vi "VisualizeCHROMADC.vi"() -> ()   [LabVIEW 2018, in "Visualization.lvlib" / "VisualizeAcPwr.lvclass"]
uses:
  VisualizeAcPwr.lvclass
  <vilib>/event_ctls.llb/usereventprio.ctl
  VisualizeBase/VisualizeBase_class/Requests/clUserEventType.ctl
  <vilib>/Utility/error.llb/Error Cluster From Error Code.vi
  <vilib>/ErrorRing/Error Ring.xnode
  VisualizeBase/VisualizeBase_class/VisualizeBase.lvclass
  <userlib>/NIST/NISTErrorLib/NISTErrorLib.lvlib
  AcPwr/AcPwrModule/AcPwrModule.lvlib
panel:
  in  "GraphAxis":u32[](array[numeric])=[0, 1, 1] max=1
  out "Chroma DC":waveform(dbl)[](graph)
  out "ErrorArray":errorcluster[](array[cluster])
  in  "QueuName":string="CHROMADCVQ"
  in  "btnStop":bool
  in  "btnReset":bool
  in  "btnClear":bool
  # "0=Left and 1=Right"
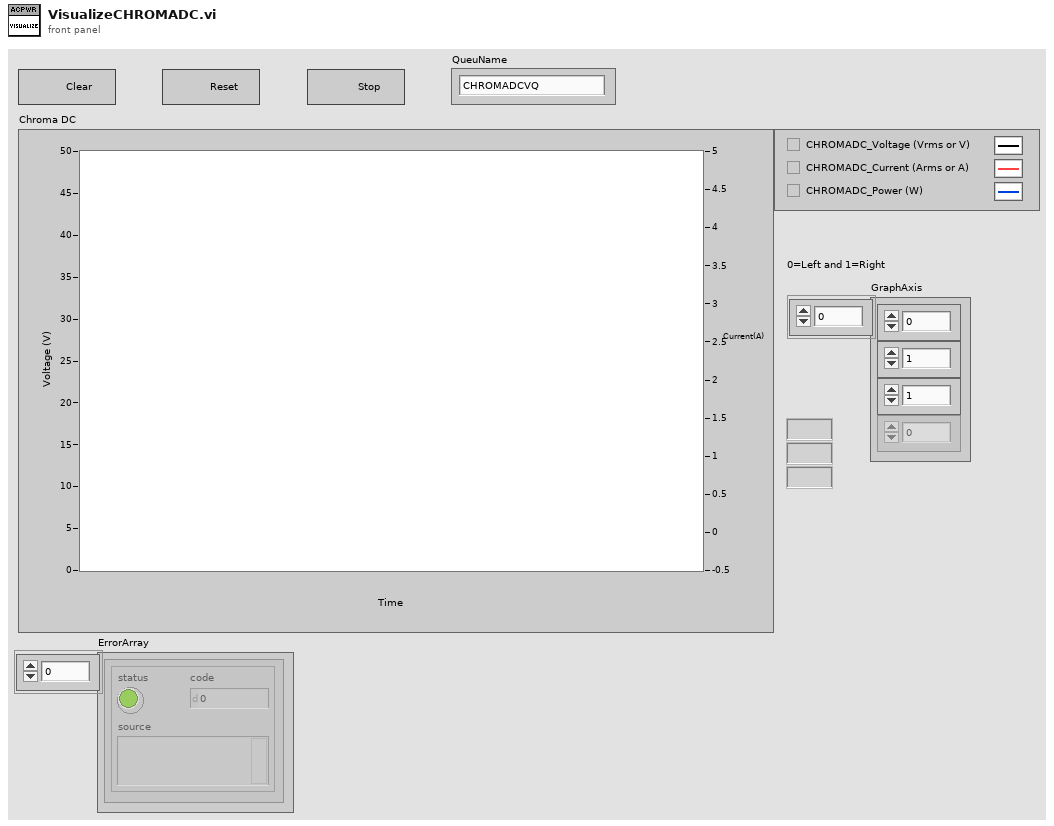
[diagram p1: front panel]
types:
  T1 = typedef "Visualization.lvlib/VisualizeBase.lvclass/clRequestEvents.ctl" = cluster{"StopRequest":refnum<user-event>, "ResetRequest":refnum<user-event>}
  T2 = typedef "AcPwrModule.lvlib/clBroadcastEvents.ctl" = cluster{"DidInit":refnum<user-event>, "StatusUpdate":refnum<user-event>, "ErrorReport":refnum<user-event>, "DidStop":refnum<user-event>, "PathToINI":refnum<user-event>, "Measurements":refnum<user-event>, "LoadConfigFile":refnum<user-event>}
  T3 = typedef "Visualization.lvlib/VisualizeBase.lvclass/clUserEventType.ctl" = cluster{"BusIndex":i8, "Data":variant}
  T4 = typedef "usereventprio.ctl" = enum32{"high priority", "normal priority"}
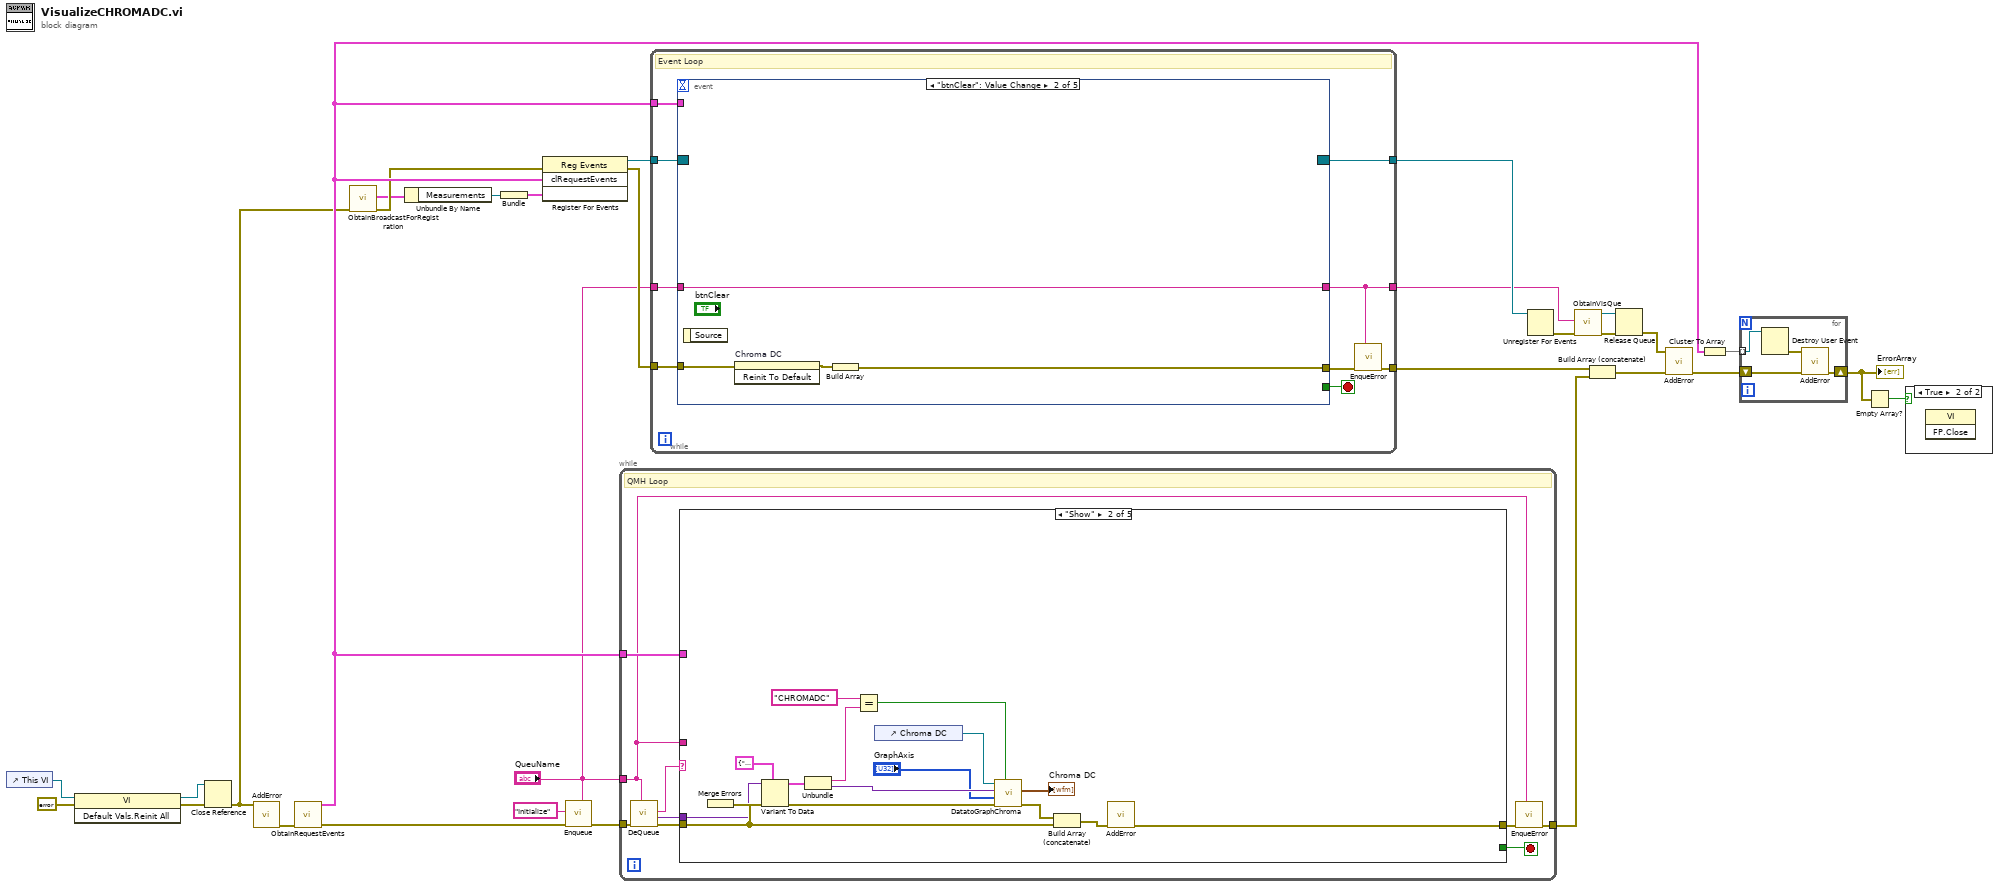
[diagram p0: block diagram]
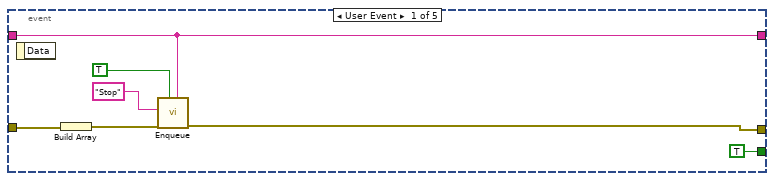
[diagram p3: hidden frame]
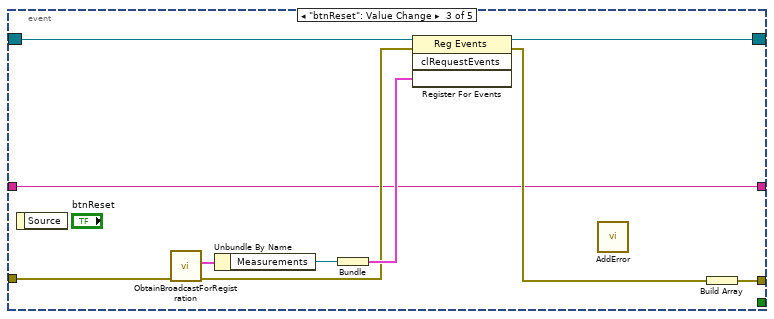
[diagram p4: hidden frame]
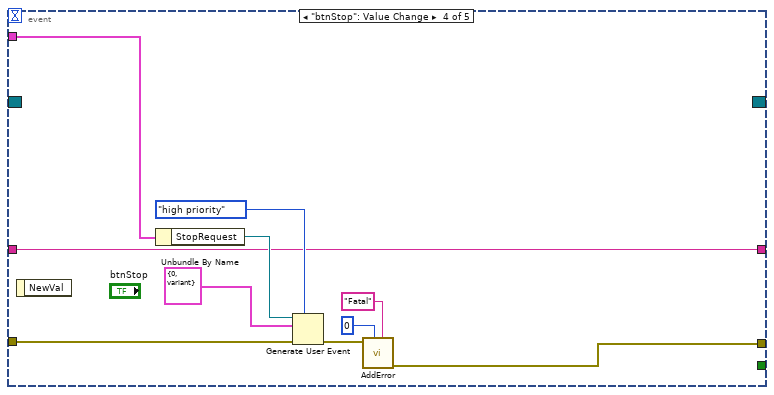
[diagram p5: hidden frame]
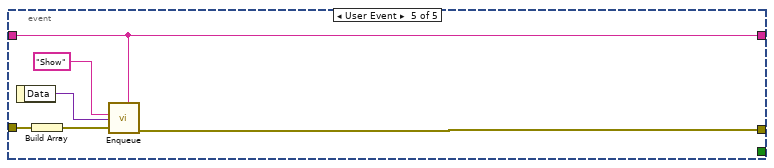
[diagram p6: hidden frame]
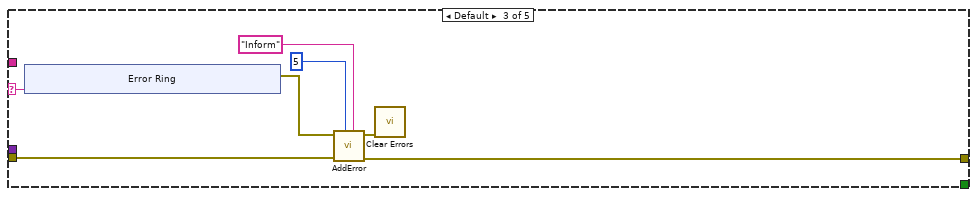
[diagram p8: hidden frame]
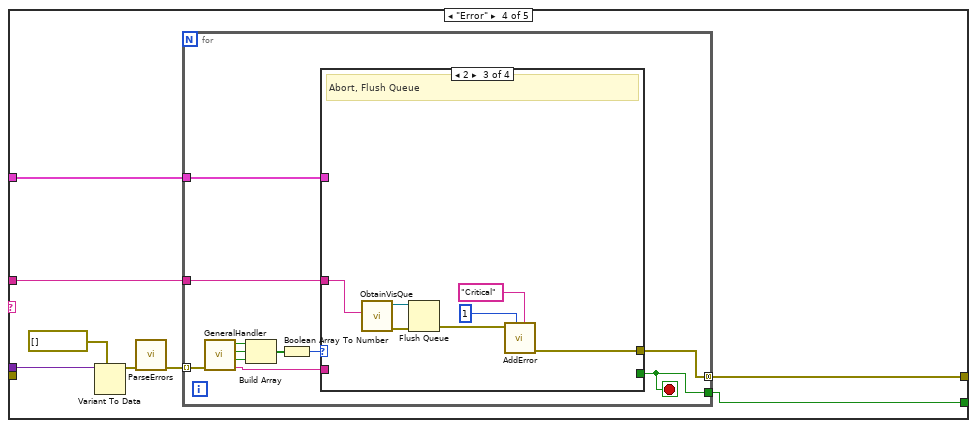
[diagram p9: hidden frame]
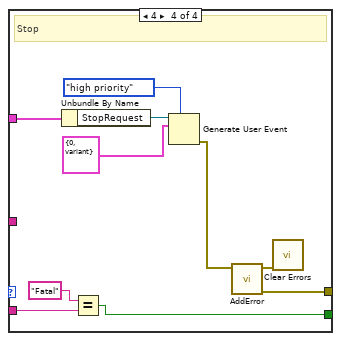
[diagram p12: hidden frame]
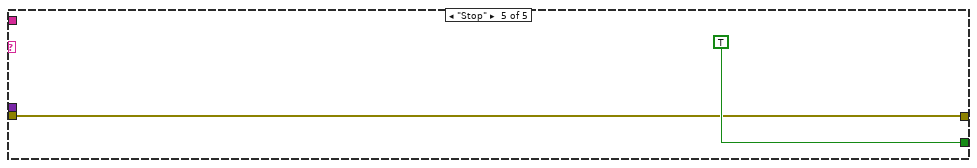
[diagram p13: hidden frame]
diagram:
  n1 = control-ref of="This VI"() -> (w10:refnum<vi>)
  n2 = invoke class="VI" method="Default Vals.Reinit All"(reference=w10, error in=errorcluster {"status"=FALSE, "code"=0, "source"=""} ("error in (no error)")) -> (reference out=w7:refnum<vi>, error out=w8:errorcluster)  [unwired: 1 in, 1 out]
  n3 = Close Reference(reference=w7, error in (no error)=w8) -> (error out=w5:errorcluster)
  n4 = call <userlib>:"AddError.vi"("error in (no error)"=w5) -> ("ErrorArray"=w27:errorcluster[])  [unwired: 9 in, 1 out]
  n5 = call "ObtainRequestEvents.vi"("Error"=w27) -> ("Error"=w12:errorcluster[], "clRequestEvents"=w16:T1)  [unwired: 9 in]
  n6 = call "ObtainBroadcastForRegistration.vi"("error in (no error)"=w5) -> ("error out"=w4:errorcluster, "clBroadcastEvents"=w3:T2)  [unwired: 9 in]
  n7 = Unbundle By Name(w3) -> ("Measurements"=w14:refnum<user-event>)
  n8 = Bundle("Measurements"=w14) -> (w13:cluster{"Measurements":refnum<user-event>})  [unwired: 1 in]
  n9 = register-events(error in=w4, w16, w13) -> (reference out=w28:refnum<event-registration>, error out=w11:errorcluster)  [unwired: 1 in]
  n10 = call "Enqueue.vi"("QueName"="QueuName", "Error"=w12, "Message"="Initialize") -> ("Error"=w29:errorcluster[])  [unwired: 8 in]
  n11 = while {
    tunnel: w29 -> [w39]
    tunnel: [w33] -> w23
    tunnel: "QueuName" -> [w31]
    tunnel: w16 -> [w32]
    stop <- w34 stop-if-true
    # "QMH Loop"
    n12 = call "DeQueue.vi"("QueName"=w31, "Error"=w39) -> ("Error"=w36:errorcluster[], "Data"=w37:variant, "Message"=w38:string)  [unwired: 7 in]
    n13 = case shown="\"Show\"" w38 {
      selector: w38 -> [_ _ w63 _ _]
      tunnel: w37 -> [_ w49 _ w78 _]
      tunnel: w36 -> [w40 w55 w61 _ w107]
      tunnel: [w40 w56 w60 w74 w107] -> w35
      tunnel: [_ _ _ w73 TRUE] -> w34
      tunnel: w32 -> [_ _ _ w72 _]
      tunnel: w31 -> [_ _ _ w71 _]
      frame "Initialize" {
      }
      frame "Show" {
        n14 = Merge Errors(w55) -> (w48:errorcluster)
        n15 = Variant To Data(error in=w48, type=cluster{string, "Data":variant} {"", "Data"=variant}, Variant=w49) -> (data=w50:cluster{string, "Data":variant}, error out=w45:errorcluster)
        n16 = Unbundle(w50) -> (w47:string, "Data"=w46:variant)
        n17 = Equal?(x="CHROMADC", y=w47) -> (x = y?=w43:bool)
        n18 = control-ref of="Chroma DC"() -> (w52:refnum<vi>)
        n19 = call "DatatoGraphChroma.vi"("Boolean"=w43, "error in (no error)"=w45, "Array 2"="GraphAxis", "Data"=w46, "WaveformChart in"=w52) -> ("error out"=w42:errorcluster, "Array"=→"Chroma DC":waveform(dbl)[])  [unwired: 3 in, 2 out]
        n20 = Build Array (concatenate)(w42, w55) -> (w54:errorcluster[])
        n21 = call <userlib>:"AddError.vi"("ErrorArray"=w54) -> ("ErrorArray"=w56:errorcluster[])  [unwired: 9 in, 1 out]
      }
      frame Default {
        n22 = xnode "Error Ring"("parameter 0"=w63) -> ("error out"=w62:errorcluster)
        n23 = call <userlib>:"AddError.vi"("Severity"="Inform" ("String"), "Priority"=u8 5, "ErrorArray"=w61, "error in (no error)"=w62) -> ("ErrorArray"=w60:errorcluster[], "error out"=w59:errorcluster)  [unwired: 6 in]
        n24 = call <vilib>:"Clear Errors.vi"("error in (no error)"=w59) -> ()  [unwired: 5 in, 2 out]
      }
      frame "Error" {
        n25 = Variant To Data(type=errorcluster[] [], Variant=w78) -> (data=w76:errorcluster[])  [unwired: 1 in, 1 out]
        n26 = call <userlib>:"ParseErrors.vi"("ErrorArray"=w76) -> ("ErrorArray"=w75:errorcluster[])  [unwired: 8 in, 2 out]
        n27 = for {
          tunnel: w75 -> [w89] mode=indexing
          tunnel: [w83] -> w74 mode=concatenating
          tunnel: [w81] -> w73
          tunnel: w72 -> [w80]
          tunnel: w71 -> [w79]
          stop <- w81 stop-if-true
          n28 = call <userlib>:"GeneralHandler.vi"("error in (no error)"=w89) -> ("Severity"=w82:string, "Stop"=w86:bool, "Abort"=w87:bool, "Continue"=w88:bool)  [unwired: 7 in]
          n29 = Build Array(w88, w87, w86) -> (w85:bool[])
          n30 = Boolean Array To Number(Boolean array=w85) -> (number=w84:u32)
          n31 = case shown="2" w84 {
            tunnel: [_ _ w94 w105] -> w83
            tunnel: w82 -> [_ _ _ w100]
            tunnel: [_ _ _ w98] -> w81
            tunnel: w80 -> [_ _ _ w97]
            tunnel: w79 -> [_ _ w90 _]
            frame 0, Default {
              # "No Dialog"
            }
            frame 1 {
              # "Continue"
            }
            frame 2 {
              # "Abort, Flush Queue"
              n32 = call "ObtainVisQue.vi"("QueName"=w90) -> ("error out"=w96:errorcluster, "queue out"=w95:refnum<queue>)  [unwired: 9 in]
              n33 = Flush Queue(queue=w95, error in (no error)=w96) -> (error out=w93:errorcluster)  [unwired: 2 out]
              n34 = call <userlib>:"AddError.vi"("Severity"="Critical" ("String"), "Priority"=u8 1, "error in (no error)"=w93) -> ("ErrorArray"=w94:errorcluster[])  [unwired: 7 in, 1 out]
            }
            frame 4 {
              # "Stop"
              n35 = Unbundle By Name(w97) -> ("StopRequest"=w106:refnum<user-event>)
              n36 = Equal?(x="Fatal", y=w100) -> (x = y?=w98:bool)
              n37 = Generate User Event(priority (normal)=usereventprio."high priority", user event=w106, event data cluster=T3 {"BusIndex"=0, "Data"=variant} ("event data")) -> (error out=w104:errorcluster)  [unwired: 1 in, 1 out]
              n38 = call <userlib>:"AddError.vi"("error in (no error)"=w104) -> ("ErrorArray"=w105:errorcluster[], "error out"=w101:errorcluster)  [unwired: 9 in]
              n39 = call <vilib>:"Clear Errors.vi"("error in (no error)"=w101) -> ()  [unwired: 5 in, 2 out]
            }
          }
        }
      }
      frame "Stop" {
      }
    }
    n40 = call "EnqueError.vi"("QueName"=w31, "Error"=w35) -> ("Error"=w33:errorcluster[])  [unwired: 9 in]
  }
  n41 = while {
    tunnel: w28 -> [w117]
    tunnel: [w114] -> w24
    tunnel: [w113] -> w26
    tunnel: w16 -> [w112]
    tunnel: w11 -> [w111]
    tunnel: "QueuName" -> [w110]
    tunnel: [w109] -> w1
    stop <- w116 stop-if-true
    # "Event Loop"
    n42 = event shown="[1] \"btnClear\": Value Change" {
      selector: w117 -> [_ _ w138 _ _]
      dyn-events: [_ _ w137 _ _] -> w113
      timeout: _ -> [_ _ _ _ _]
      tunnel: [TRUE _ _ _ _] -> w116
      tunnel: [w123 w128 w132 w146 w152] -> w115
      tunnel: w112 -> [_ _ _ w141 _]
      tunnel: w111 -> [w120 w127 w134 w140 w150]
      tunnel: w110 -> [w118 w125 w129 w139 w151]
      tunnel: [w118 w125 w129 w139 w151] -> w109
      event User Event {
        n43 = event-data() -> ()  [unwired: 1 in, 1 out]
        n44 = Build Array(w120) -> (w119:errorcluster[])
        n45 = call "Enqueue.vi"("QueName"=w118, "Priority? (F)"=TRUE, "Error"=w119, "Message"="Stop") -> ("Error"=w123:errorcluster[])  [unwired: 7 in]
      }
      event "btnClear": Value Change {
        n46 = event-data() -> ()  [unwired: 1 in, 1 out]
        n47 = invoke on="Chroma DC" class="WFChart (strict)" method="Reinit To Default"(error in=w127) -> (error out=w126:errorcluster)  [unwired: 2 in, 2 out]
        n48 = Build Array(w126) -> (w128:errorcluster[])
      }
      event "btnReset": Value Change {
        n49 = event-data() -> ()  [unwired: 1 in, 1 out]
        n50 = call "ObtainBroadcastForRegistration.vi"("error in (no error)"=w134) -> ("error out"=w131:errorcluster, "clBroadcastEvents"=w133:T2)  [unwired: 9 in]
        n51 = Unbundle By Name(w133) -> ("Measurements"=w136:refnum<user-event>)
        n52 = Bundle("Measurements"=w136) -> (w135:cluster{"Measurements":refnum<user-event>})  [unwired: 1 in]
        n53 = register-events(reference=w138, error in=w131, w135) -> (reference out=w137:refnum<event-registration>, error out=w130:errorcluster)  [unwired: 1 in]
        n54 = call <userlib>:"AddError.vi"() -> ()  [unwired: 10 in, 2 out]
        n55 = Build Array(w130) -> (w132:errorcluster[])
      }
      event "btnStop": Value Change {
        n56 = event-data() -> ()  [unwired: 1 in, 1 out]
        n57 = Unbundle By Name(w141) -> ("StopRequest"=w147:refnum<user-event>)
        n58 = Generate User Event(priority (normal)=usereventprio."high priority", user event=w147, event data cluster=T3 {"BusIndex"=0, "Data"=variant} ("event data"), error in=w140) -> (error out=w148:errorcluster)  [unwired: 1 out]
        n59 = call <userlib>:"AddError.vi"("Severity"="Fatal" ("String"), "Priority"=u8 0, "error in (no error)"=w148) -> ("ErrorArray"=w146:errorcluster[])  [unwired: 7 in, 1 out]
      }
      event User Event {
        n60 = event-data() -> ("Data"=w154:variant)  [unwired: 1 in]
        n61 = Build Array(w150) -> (w149:errorcluster[])
        n62 = call "Enqueue.vi"("QueName"=w151, "Error"=w149, "Data"=w154, "Message"="Show") -> ("Error"=w152:errorcluster[])  [unwired: 7 in]
      }
    }
    n63 = call "EnqueError.vi"("QueName"=w109, "Error"=w115) -> ("Error"=w114:errorcluster[])  [unwired: 9 in]
  }
  n64 = Unregister For Events(event registration refnum=w26) -> (error out=w22:errorcluster)  [unwired: 1 in]
  n65 = call "ObtainVisQue.vi"("error in (no error)"=w22, "QueName"=w1) -> ("error out"=w20:errorcluster, "queue out"=w19:refnum<queue>)  [unwired: 8 in]
  n66 = Build Array (concatenate)(w24, w23) -> (w21:errorcluster[])
  n67 = Release Queue(queue=w19, error in (no error)=w20) -> (error out=w18:errorcluster)  [unwired: 1 in, 2 out]
  n68 = call <userlib>:"AddError.vi"("ErrorArray"=w21, "error in (no error)"=w18) -> ("ErrorArray"=w17:errorcluster[])  [unwired: 8 in, 1 out]
  n69 = Cluster To Array(cluster=w16) -> (array=w25:refnum<user-event>[])
  n70 = for {
    tunnel: w25 -> [w158] mode=indexing
    shift-right: [w157] -> w6
    shift-left: w17 -> [w156]
    n71 = Destroy User Event(user event=w158) -> (error out=w155:errorcluster)  [unwired: 1 in]
    n72 = call <userlib>:"AddError.vi"("ErrorArray"=w156, "error in (no error)"=w155) -> ("ErrorArray"=w157:errorcluster[])  [unwired: 8 in, 1 out]
  }
  "ErrorArray" <- w6
  n73 = Empty Array?(array=w6) -> (empty?=w15:bool)
  n74 = case shown="True" w15 {
    frame False {
    }
    frame True {
      n75 = invoke class="VI" method="FP.Close"() -> ()  [unwired: 3 in, 3 out]
    }
  }
